vi "保存初始位置.vi"(10 "PosDataIn":dbl[](array[numeric]) caption="一维数据") -> ()   [LabVIEW 2018]
uses:
  Init/AllPath.vi
  <vilib>/Utility/file.llb/Write Delimited Spreadsheet (DBL).vi
panel:
  in  "文件名":string caption="请输入本次标定位置文件名"
  in  "取消":bool
  in  "确定":bool
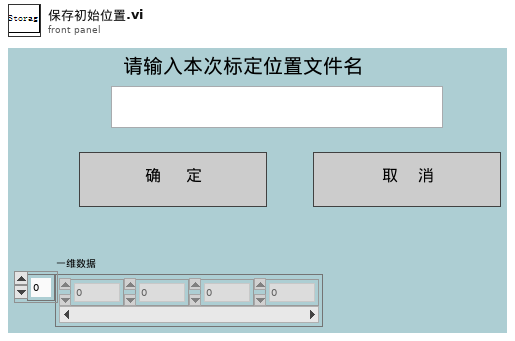
[diagram p1: front panel]
types:
  T1 = enum8{"Enabled", "Disabled", "Disabled and Grayed Out"}
  T2 = cluster{"能量/功率":path, " 示波器":path, " 光谱仪":path, "偏振":path, "近远场":cluster{" 近场图片":path, " 远场图片":path, "发散角数据":path}, "参数":path, " 基路径":path, "文件名信息":path, "输出模板路径":path, "输出报告路径":path}
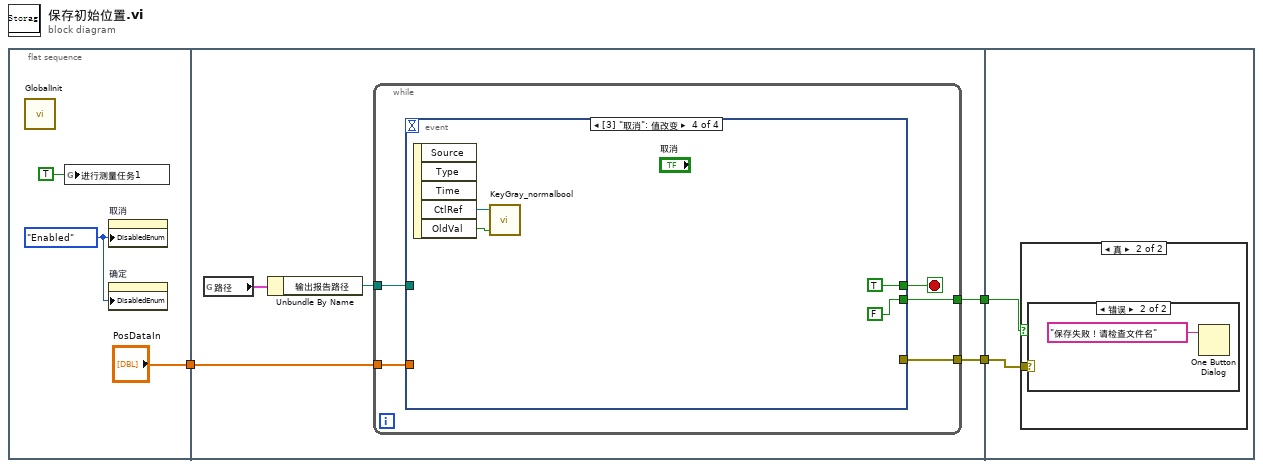
[diagram p0: block diagram]
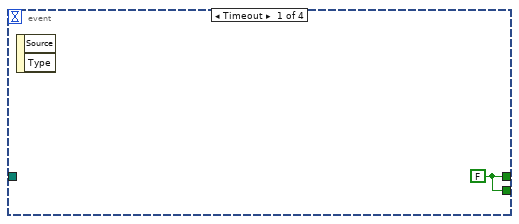
[diagram p2: hidden frame]
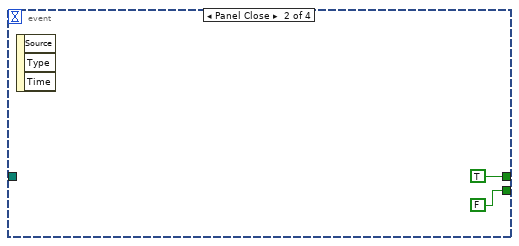
[diagram p3: hidden frame]
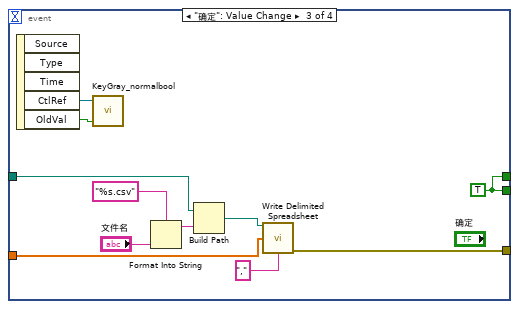
[diagram p4: hidden frame]
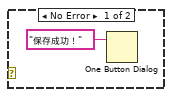
[diagram p6: hidden frame]
diagram:
  n1 = flat-sequence {
    tunnel: ["PosDataIn"] -> w3
    tunnel: w3 -> [w9]
    tunnel: [w8] -> w2
    tunnel: [w7] -> w1
    tunnel: w2 -> [w36]
    tunnel: w1 -> [w35]
    frame #0 {
      w6 = T1."Enabled" ("禁用")
      n2 = call "GlobalInit.vi"() -> ()  [unwired: 1 in, 1 out]
      n3 = global write "参数.vi" "进行测量任务1"(TRUE ("是否完成本次测量？")) -> ()
      n4 = property on="取消" class="Bool (严格)"("DisabledEnum"=w6) -> ()  [unwired: 2 in, 2 out]
      n5 = property on="确定" class="Bool (严格)"("DisabledEnum"=w6) -> ()  [unwired: 2 in, 2 out]
    }
    frame #1 {
      n6 = global read "AllPath.vi" "路径"() -> (w11:T2)
      n7 = Unbundle By Name(w11) -> ("输出报告路径"=w10:path)
      n8 = while {
        tunnel: [w15] -> w7
        tunnel: w10 -> [w14]
        tunnel: w9 -> [w13]
        tunnel: [w12] -> w8
        stop <- w16 stop-if-true
        n9 = event shown="[3] \"取消\": 值改变" {
          selector: _ -> [_ _ _ _]
          dyn-events: _ -> [_ _ _ _]
          timeout: _ -> [_ _ _ _]
          tunnel: [w17 TRUE w21 TRUE] -> w16
          tunnel: [w17 FALSE w21 FALSE] -> w15
          tunnel: w14 -> [_ _ w25 _]
          tunnel: w13 -> [_ _ w22 _]
          tunnel: [_ _ w20 _] -> w12
          event Timeout {
            w17 = FALSE
            n10 = event-data() -> ()  [unwired: 1 in, 2 out]
          }
          event Panel Close {
            n11 = event-data() -> ()  [unwired: 1 in, 3 out]
          }
          event "确定": Value Change {
            w21 = TRUE
            n12 = event-data() -> ("CtlRef"=w30:refnum<vi>, "OldVal"=w29:bool)  [unwired: 1 in, 3 out]
            n13 = call "KeyGray_normalbool.vi"("OldVal"=w29, "引用"=w30) -> ()  [unwired: 2 in]
            n14 = Format Into String(format string="%s.csv" ("格式字符串"), "文件名") -> (resulting string=w24:string)  [unwired: 2 in, 1 out]
            n15 = Build Path(base path=w25, name or relative path=w24) -> (appended path=w23:path)
            n16 = call-poly <vilib>:"Write Delimited Spreadsheet.vi"("file path (dialog if empty)"=w23, "1D data"=w22, "delimiter (\\t)"="," ("delimiter (\\t)")) -> ("error out"=w20:errorcluster)  [unwired: 11 in, 1 out]
          }
          event "取消": Value Change {
            n17 = event-data() -> ("CtlRef"=w33:refnum<vi>, "OldVal"=w32:bool)  [unwired: 1 in, 3 out]
            n18 = call "KeyGray_normalbool.vi"("OldVal"=w32, "引用"=w33) -> ()  [unwired: 2 in]
          }
        }
      }
    }
    frame #2 {
      n19 = case shown="真" w35 {
        tunnel: w36 -> [_ w37]
        frame False {
        }
        frame True {
          n20 = case shown="错误" w37 {
            frame No Error {
              n21 = One Button Dialog(message="保存成功！" ("消息")) -> ()  [unwired: 1 in, 1 out]
            }
            frame Error {
              n22 = One Button Dialog(message="保存失败！请检查文件名" ("消息")) -> ()  [unwired: 1 in, 1 out]
            }
          }
        }
      }
    }
  }
